vi "Save Data.vi"(8 "error in (no error)":errorcluster, 9 ">> Save Data? >>":bool, 10 "U16 Array":u16[][][](array[numeric]), 11 "Byte Stream File in":refnum<file>) -> (0 "error out":errorcluster)   [LabVIEW 2015, in "Intensity Processing.lvclass"]
uses:
  Intensity/Intensity Processing.lvclass
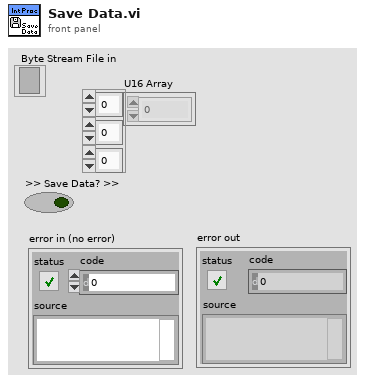
[diagram p1: front panel]
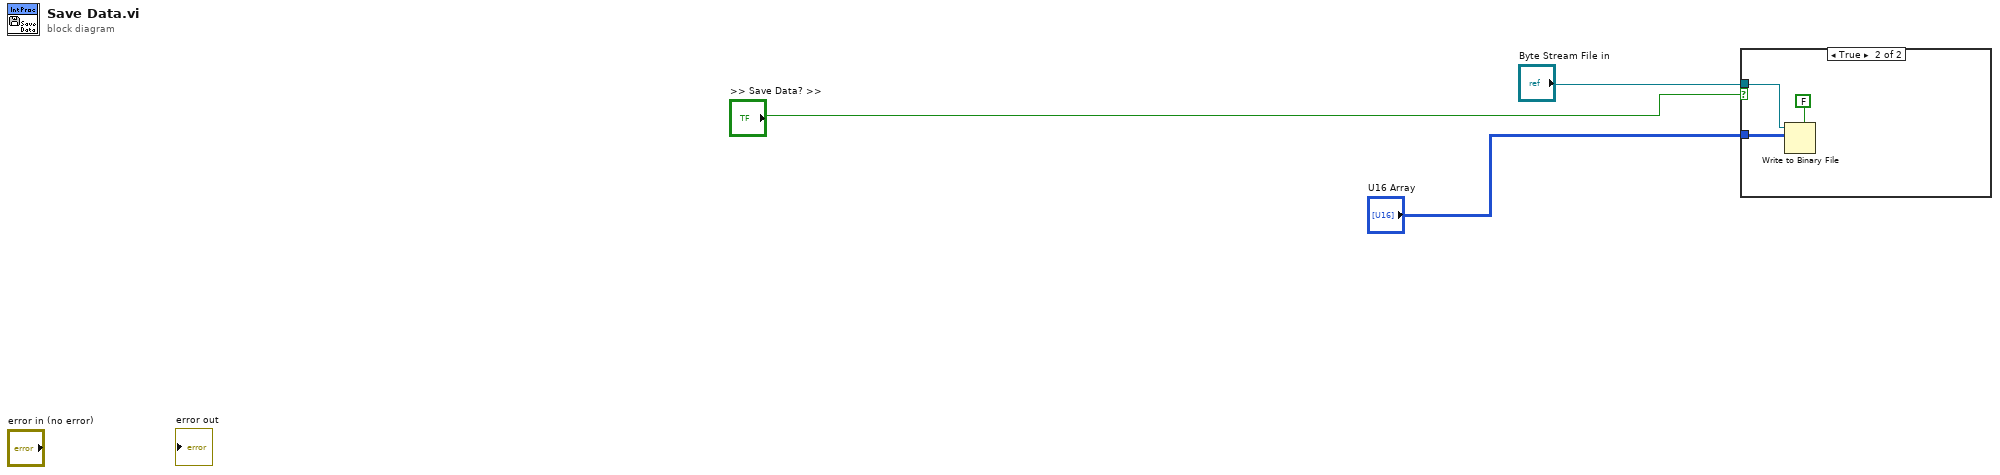
[diagram p0: block diagram]
diagram:
  n1 = case shown="True" ">> Save Data? >>" {
    tunnel: "U16 Array" -> [_ w5]
    tunnel: "Byte Stream File in" -> [_ w4]
    frame False {
    }
    frame True {
      n2 = Write to Binary File(file (use dialog)=w4, data=w5, 5:FALSE ("prepend array or string size? (T)")) -> ()  [unwired: 3 in, 3 out]
    }
  }
